vi "provide_note_book_info.vi"(8 "error in (no error)":errorcluster, 10 "notebook string in":string, 11 "GenericDataCollection in":refnum<class "GenericDataCollection.lvclass">) -> (0 "error out":errorcluster, 2 "notebook string out":string, 3 "GenericDataCollection out":refnum<class "GenericDataCollection.lvclass">)   [LabVIEW 2010, in "GenericDataCollection.lvclass"]
uses:
  GenericDataCollection.lvclass
  common/classes/GenericComponent/GenericComponent/class_data.vi
  ImagingMode/GenericImagingMode/GenericImagingMode/GenericImagingMode.lvclass
  ScanHead/GenericScanHead/GenericScanHead/GenericScanHead.lvclass
  Stimulator/GenericStimulator/GenericStimulator/GenericStimulator.lvclass
  common/classes/GenericComponent/GenericComponent/GenericComponent.lvclass
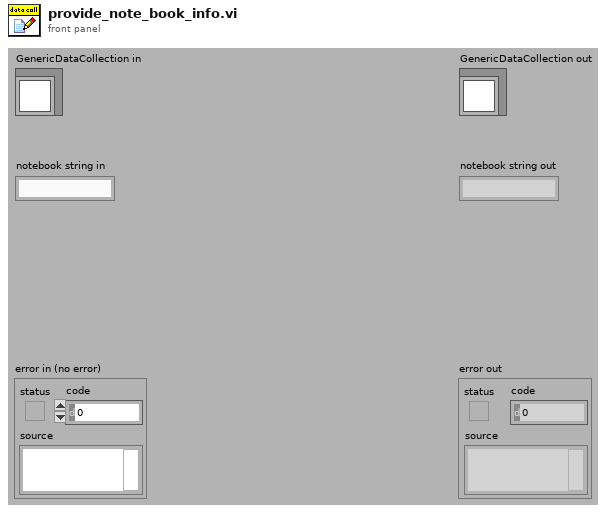
[diagram p1: front panel]
types:
  T1 = typedef "run_mode_enum.ctl" = enum16{"focus mode", "single sweep mode", "experiment mode"}
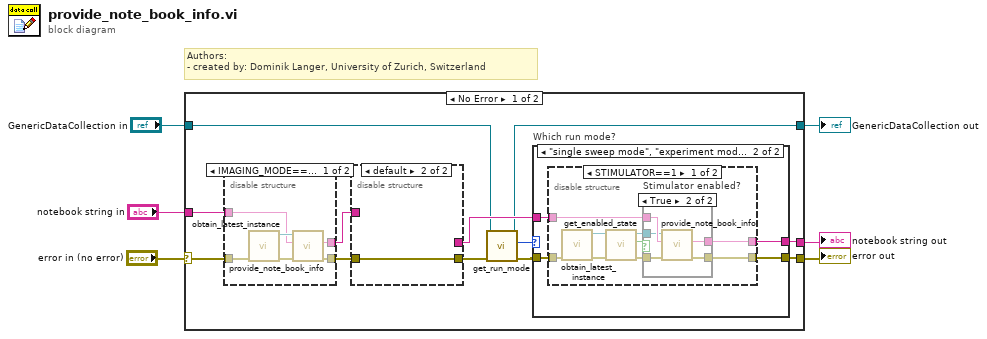
[diagram p0: block diagram]
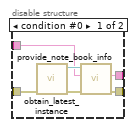
[diagram p5: hidden frame]
diagram:
  # "Authors: \n- created by: Dominik Langer, University of Zurich, Switzerland"
  n1 = case shown="No Error" "error in (no error)" {
    selector: "error in (no error)" -> [w18 w59]
    tunnel: [w11 w59] -> w5
    tunnel: "GenericDataCollection in" -> [w8 w58]
    tunnel: [w7 w58] -> w3
    tunnel: "notebook string in" -> [w17 w57]
    tunnel: [w10 w57] -> w1
    frame No Error {
      n2 = disable-structure shown="IMAGING_MODE==1" {
        disable-tunnel: w18 -> [w55 w56]
        disable-tunnel: [w52 w56] -> w16
        disable-tunnel: w17 -> [w51 _]
        disable-tunnel: [w50 _] -> w15
        frame condition #0 {
          n3 = call "obtain_latest_instance.vi"("error in (no error)"=w55) -> ("error out"=w54:errorcluster, "GenericScanMode out"=w53:refnum<class "GenericImagingMode.lvclass">)  [unwired: 9 in]
          n4 = call-dynamic "provide_note_book_info.vi"("error in (no error)"=w54, "notebook string in"=w51, "GenericPlugin in"=w53) -> ("error out"=w52:errorcluster, "notebook string out"=w50:string)  [unwired: 6 in, 1 out]
        }
        frame condition #1 (active) {
        }
      }
      n5 = disable-structure shown="default" {
        disable-tunnel: w16 -> [w48 w49]
        disable-tunnel: [w45 w49] -> w12
        disable-tunnel: w15 -> [w44 _]
        disable-tunnel: [w43 _] -> w9
        frame condition #0 {
          n6 = call "obtain_latest_instance.vi"("error in (no error)"=w48) -> ("error out"=w47:errorcluster, "GenericScanHead out"=w46:refnum<class "GenericScanHead.lvclass">)  [unwired: 9 in]
          n7 = call-dynamic "provide_note_book_info.vi"("error in (no error)"=w47, "notebook string in"=w44, "GenericPlugin in"=w46) -> ("error out"=w45:errorcluster, "notebook string out"=w43:string)  [unwired: 6 in, 1 out]
        }
        frame condition #1 (active) {
        }
      }
      n8 = call "get_run_mode.vi"("error in (no error)"=w12, "GenericPlugin in"=w8) -> ("error out"=w13:errorcluster, "run mode"=w14:T1, "GenericPlugin out"=w7:refnum<class "GenericDataCollection.lvclass">)  [unwired: 5 in, 2 out]
      n9 = case "Which run mode?" shown="\"single sweep mode\", \"experiment mode\"" w14 {
        tunnel: w9 -> [w20 w24]
        tunnel: [w19 w23] -> w11
        tunnel: [w20 w22] -> w10
        tunnel: w13 -> [w19 w21]
        frame Default {
        }
        frame "single sweep mode", "experiment mode" {
          n10 = disable-structure shown="STIMULATOR==1" {
            disable-tunnel: w21 -> [w33 w42]
            disable-tunnel: [w32 w42] -> w23
            disable-tunnel: w24 -> [w31 w41]
            disable-tunnel: [w30 w41] -> w22
            frame condition #0 {
              n11 = call "obtain_latest_instance.vi"("error in (no error)"=w33) -> ("error out"=w29:errorcluster, "GenericStimulator out"=w27:refnum<class "GenericStimulator.lvclass">)  [unwired: 9 in]
              n12 = call-dynamic "get_enabled_state.vi"("error in (no error)"=w29, "GenericStimulator in"=w27) -> ("error out"=w28:errorcluster, "stimulator enabled?"=w25:bool, "GenericStimulator out"=w26:refnum<class "GenericStimulator.lvclass">)  [unwired: 7 in]
              n13 = case "Stimulator enabled?" shown="True" w25 {
                tunnel: [w35 w40] -> w32
                tunnel: w31 -> [w34 w39]
                tunnel: [w34 w38] -> w30
                tunnel: w28 -> [w35 w37]
                tunnel: w26 -> [_ w36]
                frame False {
                }
                frame True {
                  n14 = call-dynamic "provide_note_book_info.vi"("error in (no error)"=w37, "notebook string in"=w39, "GenericPlugin in"=w36) -> ("error out"=w40:errorcluster, "notebook string out"=w38:string)  [unwired: 6 in, 1 out]
                }
              }
            }
            frame condition #1 (active) {
            }
          }
        }
      }
    }
    frame Error {
    }
  }
  "error out" <- w5
  "GenericDataCollection out" <- w3
  "notebook string out" <- w1
